vi "read file.vi"(0 "reference in":refnum<class "TDMS_DataHandler.lvclass">, 5 "error in (no error)":errorcluster) -> (14 "reference out":refnum<class "TDMS_DataHandler.lvclass">, 15 "Channel name(s)":string[](array[string]), 16 "Data out":waveform(dbl)[](array[waveform]), 17 "Group name out":string[](array[string]), 19 "error out":errorcluster)   [LabVIEW 2019, in "TDMS_DataHandler.lvclass"]
uses:
  TDMS_DataHandler.lvclass
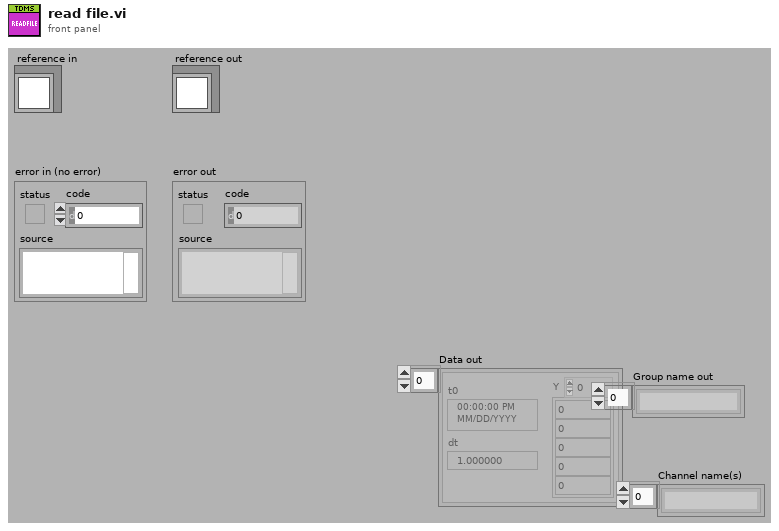
[diagram p1: front panel]
types:
  T1 = typedef "TDMS_DataHandler.lvclass/ObjectAttributes.ctl" = cluster{"Directory":path, "FilePath":path, "FileRef":refnum<k34>, "ExperimentName":string, "GroupName":string, "ChannelNames":string[], "Datum":waveform(dbl)[], "Group_Metadata":cluster{"property names":string[], "property values":variant[]}, "Channel_Metadata":cluster{"property names":string[], "property values":variant[]}}
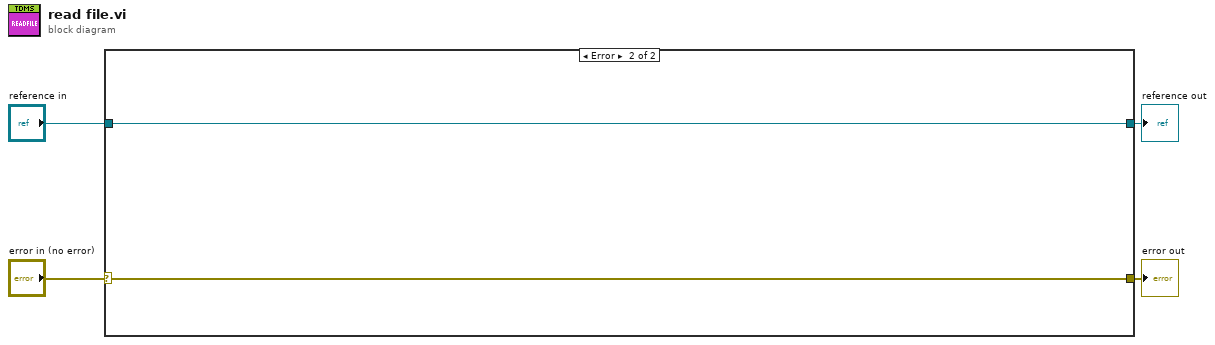
[diagram p0: block diagram]
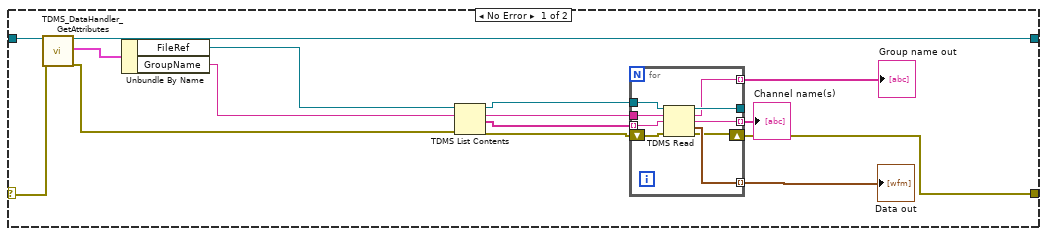
[diagram p2: hidden frame]
diagram:
  n1 = case shown="Error" "error in (no error)" {
    selector: "error in (no error)" -> [w17 w30]
    tunnel: [w9 w30] -> w3
    tunnel: [w18 w29] -> w1
    tunnel: "reference in" -> [w19 w29]
    frame No Error {
      n2 = call "TDMS_DataHandler_GetAttributes.vi"("reference in"=w19, "error in (no error)"=w17) -> ("reference out"=w18:refnum<class "TDMS_DataHandler.lvclass">, "attributes"=w16:T1, "error out"=w8:errorcluster)  [unwired: 14 in, 1 out]
      n3 = Unbundle By Name(w16) -> ("FileRef"=w7:refnum<k34>, "GroupName"=w6:string)
      n4 = TDMS List Contents(4:w8, 6:w6, 7:w7) -> (0:w12:errorcluster, 1:w14:string[], 2:w15:string, 3:w13:refnum<k34>)
      n5 = for {
        tunnel: [w28] -> _
        tunnel: w15 -> [w27]
        tunnel: w14 -> [w26] mode=indexing
        tunnel: w13 -> [w25]
        tunnel: [w23] -> w10 mode=indexing
        tunnel: [w22] -> w11 mode=indexing
        shift-right: [w21] -> w9
        shift-left: w12 -> [w24]
        tunnel: [w20] -> w5 mode=indexing
        n6 = TDMS Read(0:w25, 5:w27, 7:w26, 11:w24) -> (4:w28:refnum<k34>, 6:w23:string, 8:w20:string, 10:w22:waveform(dbl), 15:w21:errorcluster)  [unwired: 4 in, 1 out]
      }
      "Data out" <- w11
      "Group name out" <- w10
      "Channel name(s)" <- w5
    }
    frame Error {
    }
  }
  "error out" <- w3
  "reference out" <- w1
